vi "fan.vi"(11 "Shared_strings":string[][](array[string])) -> ()   [LabVIEW 2018]
uses:
  Global Variables.vi
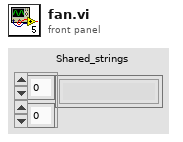
[diagram p1: front panel]
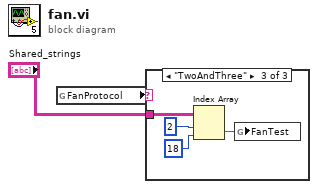
[diagram p0: block diagram]
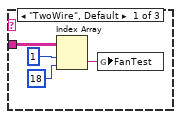
[diagram p2: hidden frame]
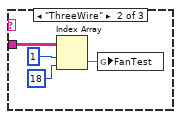
[diagram p3: hidden frame]
diagram:
  n1 = global read "Global Variables.vi" "FanProtocol"() -> (w1:string)
  n2 = case shown="\"TwoAndThree\"" w1 {
    tunnel: "Shared_strings" -> [w6 w7 w11]
    frame "TwoWire", Default {
      n3 = Index Array(array=w6, index (row)=1, index (col)=18) -> (element=w3:string)
      n4 = global write "Global Variables.vi" "FanTest"(w3) -> ()
    }
    frame "ThreeWire" {
      n5 = Index Array(array=w7, index (row)=1, index (col)=18) -> (element=w8:string)
      n6 = global write "Global Variables.vi" "FanTest"(w8) -> ()
    }
    frame "TwoAndThree" {
      n7 = Index Array(array=w11, index (row)=2, index (col)=18) -> (element=w12:string)
      n8 = global write "Global Variables.vi" "FanTest"(w12) -> ()
    }
  }
